vi "rgb2labBu1.vi"(0 "R":u8[][](array[numeric]), 2 "G":u8[][](array[numeric]), 5 "B":u8[][](array[numeric])) -> (1 "hang":i32, 4 "lie":i32, 6 "LZ":dbl[](array[numeric]), 7 "aZ":dbl[](array[numeric]), 8 "bZ":dbl[](array[numeric]))   [LabVIEW 2018]
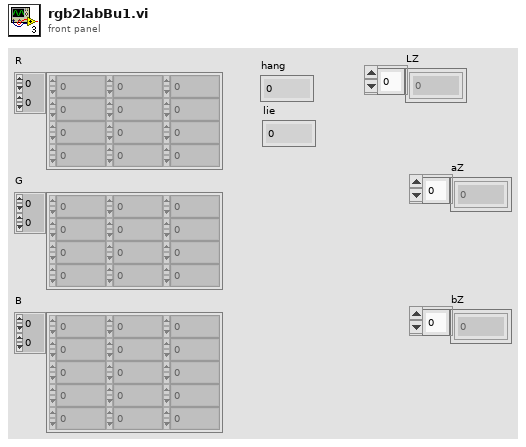
[diagram p1: front panel]
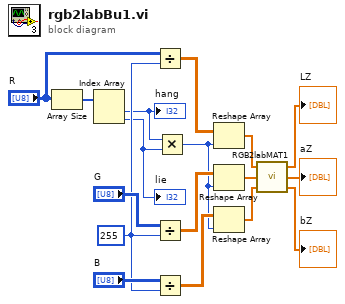
[diagram p0: block diagram]
diagram:
  w15 = 255
  n1 = Array Size(array="R") -> (size(s)=w14:i32[])
  n2 = Index Array(array=w14) -> (element #1=w8:i32, element #2=w7:i32)  [unwired: 2 in]
  "hang" <- w8
  "lie" <- w7
  n3 = Divide(x="R", y=w15) -> (x/y=w11:dbl[][])
  n4 = Divide(x="G", y=w15) -> (x/y=w12:dbl[][])
  n5 = Divide(x="B", y=w15) -> (x/y=w10:dbl[][])
  n6 = Multiply(x=w8, y=w7) -> (x*y=w9:i32)
  n7 = Reshape Array(w11, w9) -> (w6:dbl[])
  n8 = Reshape Array(w12, w9) -> (w5:dbl[])
  n9 = Reshape Array(w10, w9) -> (w4:dbl[])
  n10 = call "RGB2labMAT1.vi"(3:"sRL"=w4, "sGL"=w5, 5:"sRL"=w6) -> ("b"=→"bZ":dbl[], "a"=→"aZ":dbl[], "L"=→"LZ":dbl[])
